vi "MatrixInit.vi"() -> ()   [LabVIEW 2026]
uses:
  <vilib>/MakerHub/LINX/Private/Type Defs/Peripherals/SPI/SPI Configuration.ctl
  <vilib>/MakerHub/LINX/Private/Type Defs/Peripherals/SPI/SPI Bit Order.ctl
  <vilib>/MakerHub/LINX/Private/Type Defs/Peripherals/SPI/SPI Mode.ctl
  <vilib>/MakerHub/LINX/Public/Peripherals/SPI/SPI Write Read N Frames.vi
  <vilib>/MakerHub/LINX/Private/Local IO/LinxSpiWriteRead.vi
  <vilib>/MakerHub/LINX/Public/Utilities/Check Channel.vi
  <vilib>/MakerHub/LINX/Private/Utilties/Generate Error.vi
  <vilib>/MakerHub/LINX/Public/Utilities/Open Serial.vi
  <vilib>/MakerHub/LINX/LMH-LINX.lvlib
  <vilib>/MakerHub/LINX/Private/Type Defs/Peripherals/SPI/SPI CS Logic Level.ctl
  <vilib>/MakerHub/LINX/Public/Peripherals/SPI/SPI CS Config.ctl
panel:
  in  "CS Configuration":T1
  out "Data":u8
  out "Address":u8
  out "Array 2":u8[](array[numeric])
  in  "Array":bool[][](array[boolean])
  in  "Stop Button":bool
  in  "SPI Configuration":T3={"Clock Frequency"=1000000, "Bit Order"=enum."LSb First", "SPI Mode"=enum."Mode 0"}
  in  "Serial Port":refnum<visa-resource-name>="N/A"
  # "Default 1000000 Hz"
  # "MAX7219 Matrix requires Most Significant Bit (MSb)!"
  # "Specify CS Pin on Arduino (10 in our setup)"
  # "MAX7219 requires Active Low Chip Select!"
  # "Just for debugging purposes!"
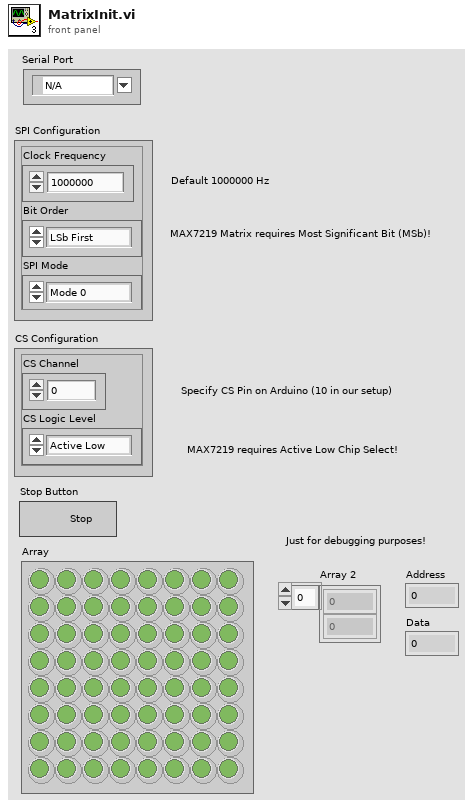
[diagram p1: front panel]
types:
  T1 = typedef "LMH-LINX.lvlib/SPI CS Config.ctl" = cluster{"CS Channel":u8, "CS Logic Level":T2}
  T2 = typedef "LMH-LINX.lvlib/SPI CS Logic Level.ctl" = enum8{"Active Low", "Active High"}
  T3 = typedef "LMH-LINX.lvlib/SPI Configuration.ctl" = cluster{"Clock Frequency":u32, "Bit Order":T4, "SPI Mode":T5}
  T4 = typedef "LMH-LINX.lvlib/SPI Bit Order.ctl" = enum8{"LSb First", "MSb First"}
  T5 = typedef "LMH-LINX.lvlib/SPI Mode.ctl" = enum8{"Mode 0", "Mode 1", "Mode 2", "Mode 3"}
  T6 = typedef "LMH-LINX.lvlib/LINX Ref.ctl" = cluster{"IO":T7, "Interface":T8, "LINX Device Config":T9}
  T7 = typedef "LMH-LINX.lvlib/Platform.ctl" = enum16{"Remote", "Local"}
  T8 = typedef "LMH-LINX.lvlib/Interface.ctl" = enum16{"Serial", "TCP"}
  T9 = typedef "LMH-LINX.lvlib/Device.lvlib/LINX Device Config.ctl" = cluster{"Interface":T8, "COM Port":refnum<visa-resource-name>, "TCP Configuration":T10, "Device Family":u8, "Device ID":u8, "Device Name":string, "TCP Ref":refnum<k5>, "Channels":T11}
  T10 = typedef "LMH-LINX.lvlib/Device.lvlib/TCP Config.ctl" = cluster{"IP Address":string, "Port":u16}
  T11 = typedef "LMH-LINX.lvlib/Channels.ctl" = cluster{"DI":u8[], "DO":u8[], "AI":u8[], "AO":u8[], "PWM":u8[], "QE":u8[], "UART":u8[], "I2C 2":u8[], "SPI":u8[], "CAN":u8[], "Servo":u8[], "AI Ref (V)":dbl, "AI Resolution (Bits)":u8, "AO Ref (V)":dbl, "AO Resolution (Bits)":u8}
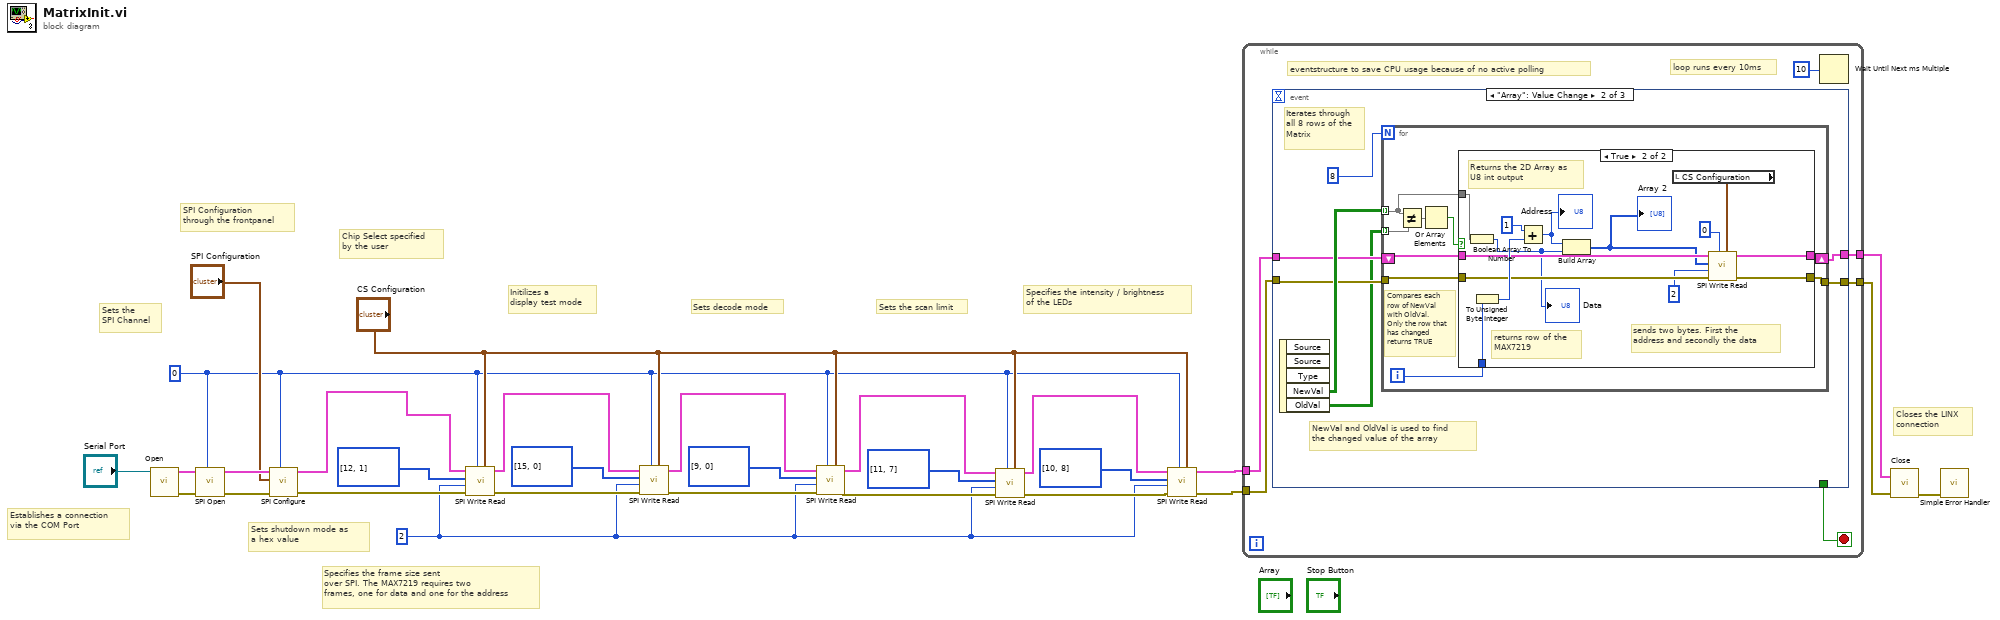
[diagram p0: block diagram]
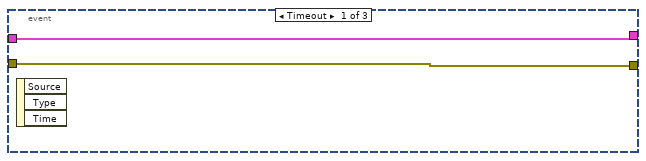
[diagram p2: hidden frame]
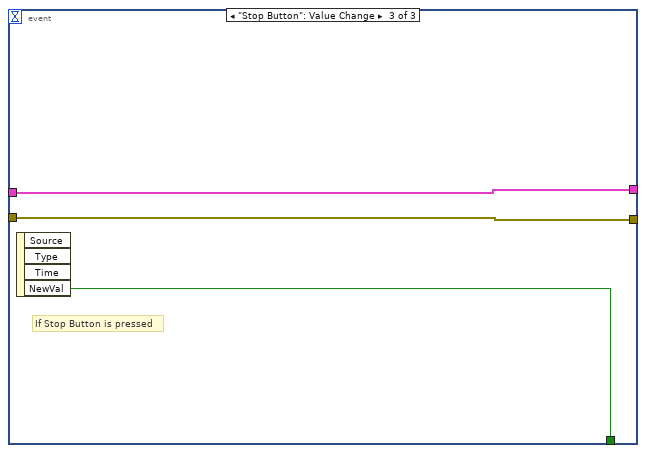
[diagram p4: hidden frame]
diagram:
  w2 = u8 2 ("SPI Frame Size")
  w1 = u8 0 ("SPI Channel (0)")
  # "Closes the LINX\nconnection"
  # "Specifies the intensity / brightness\nof the LEDs"
  # "Sets the scan limit"
  # "Sets decode mode"
  # "Initilizes a\ndisplay test mode"
  # "Sets shutdown mode as \na hex value"
  # "Specifies the frame size sent\nover SPI. The MAX7219 requires two\nframes, one for data and one for the address"
  # "Chip Select specified\nby the user"
  # "SPI Configuration\nthrough the frontpanel"
  # "Establishes a connection via the COM Port"
  # "Sets the\nSPI Channel"
  n1 = call-poly <vilib>:"Open.vi"("Serial Port"="Serial Port") -> ("Error Out"=w26:errorcluster, "LINX Resource"=w27:T6)  [unwired: 8 in, 1 out]
  n2 = call <vilib>:"SPI Open.vi"("SPI Channel (0)"=w1, "Error In"=w26, "LINX Resource"=w27) -> ("Error Out"=w24:errorcluster, "LINX Resource"=w25:T6)  [unwired: 7 in]
  n3 = call <vilib>:"SPI Configure.vi"("SPI Channel (0)"=w1, "Error In"=w24, "SPI Configuration"="SPI Configuration", "LINX Resource"=w25) -> ("Error Out"=w4:errorcluster, "LINX Resource"=w3:T6)  [unwired: 5 in, 1 out]
  n4 = call-poly <vilib>:"SPI Write Read.vi"("CS Configuration"="CS Configuration", "SPI Channel (0)"=w1, "Error In"=w4, "SPI Frame Size"=w2, "Data"=u8[] [12, 1], "LINX Resource"=w3) -> ("Error Out"=w15:errorcluster, "LINX Resource"=w14:T6)  [unwired: 2 in, 2 out]
  n5 = call-poly <vilib>:"SPI Write Read.vi"("CS Configuration"="CS Configuration", "SPI Channel (0)"=w1, "Error In"=w15, "SPI Frame Size"=w2, "Data"=u8[] [15, 0], "LINX Resource"=w14) -> ("Error Out"=w13:errorcluster, "LINX Resource"=w12:T6)  [unwired: 2 in, 2 out]
  n6 = call-poly <vilib>:"SPI Write Read.vi"("CS Configuration"="CS Configuration", "SPI Channel (0)"=w1, "Error In"=w13, "SPI Frame Size"=w2, "Data"=u8[] [9, 0], "LINX Resource"=w12) -> ("Error Out"=w10:errorcluster, "LINX Resource"=w11:T6)  [unwired: 2 in, 2 out]
  n7 = call-poly <vilib>:"SPI Write Read.vi"("CS Configuration"="CS Configuration", "SPI Channel (0)"=w1, "Error In"=w10, "SPI Frame Size"=w2, "Data"=u8[] [11, 7], "LINX Resource"=w11) -> ("Error Out"=w8:errorcluster, "LINX Resource"=w9:T6)  [unwired: 2 in, 2 out]
  n8 = call-poly <vilib>:"SPI Write Read.vi"("CS Configuration"="CS Configuration", "SPI Channel (0)"=w1, "Error In"=w8, "SPI Frame Size"=w2, "Data"=u8[] [10, 8], "LINX Resource"=w9) -> ("Error Out"=w6:errorcluster, "LINX Resource"=w5:T6)  [unwired: 2 in, 2 out]
  n9 = while {
    tunnel: w6 -> [w32]
    tunnel: w5 -> [w34]
    tunnel: [w33] -> w22
    tunnel: [w31] -> w21
    stop <- w30 stop-if-true
    # "loop runs every 10ms"
    # "eventstructure to save CPU usage because of no active polling"
    n10 = event shown="[1] \"Array\": Value Change" {
      selector: _ -> [_ _ _]
      dyn-events: _ -> [_ _ _]
      timeout: _ -> [_ _ _]
      tunnel: w34 -> [w37 w43 w72]
      tunnel: [w37 w42 w72] -> w33
      tunnel: w32 -> [w36 w41 w71]
      tunnel: [w36 w40 w71] -> w31
      tunnel: [_ _ w70] -> w30
      event Timeout {
        n11 = event-data() -> ()  [unwired: 1 in, 3 out]
      }
      event "Array": Value Change {
        # "Iterates through\nall 8 rows of the\nMatrix"
        # "NewVal and OldVal is used to find\nthe changed value of the array"
        n12 = event-data() -> ("NewVal"=w44:bool[][], "OldVal"=w38:bool[][])  [unwired: 1 in, 3 out]
        n13 = for {
          N: 8 -> [_]
          tunnel: w44 -> [w45] mode=indexing
          shift-right: [w50] -> w42
          shift-left: w43 -> [w52]
          tunnel: w41 -> [w51]
          tunnel: [w49] -> w40
          tunnel: w38 -> [w48] mode=indexing
          i -> [w53]
          # "Compares each row of NewVal with OldVal.\nOnly the row that has changed returns TRUE"
          n14 = Not Equal?(x=w45, y=w48) -> (x != y?=w47:bool[])
          n15 = Or Array Elements(Boolean array=w47) -> (logical OR=w46:bool)
          n16 = case shown="True" w46 {
            tunnel: w53 -> [_ w68]
            tunnel: w52 -> [w55 w64]
            tunnel: w51 -> [w54 w63]
            tunnel: [w55 w62] -> w50
            tunnel: [w54 w61] -> w49
            tunnel: w45 -> [_ w57]
            frame False {
            }
            frame True {
              # "returns row of the\nMAX7219"
              # "sends two bytes. First the\naddress and secondly the data"
              # "Returns the 2D Array as\nU8 int output"
              n17 = Boolean Array To Number(Boolean array=w57) -> (number=w58:u8)
              "Data" <- w58
              n18 = To Unsigned Byte Integer(number=w68) -> (unsigned 8bit integer=w67:u8)
              n19 = Add(x=u8 1 ("y"), y=w67) -> (x+y=w59:u8)
              "Address" <- w59
              n20 = Build Array(w59, w58) -> (w60:u8[])
              "Array 2" <- w60
              n21 = local read "CS Configuration"() -> (w65:T1)
              n22 = call-poly <vilib>:"SPI Write Read.vi"("CS Configuration"=w65, "SPI Channel (0)"=u8 0, "Error In"=w63, "SPI Frame Size"=u8 2, "Data"=w60, "LINX Resource"=w64) -> ("Error Out"=w61:errorcluster, "LINX Resource"=w62:T6)  [unwired: 2 in, 2 out]
            }
          }
        }
      }
      event "Stop Button": Value Change {
        # "If Stop Button is pressed"
        n23 = event-data() -> ("NewVal"=w70:bool)  [unwired: 1 in, 3 out]
      }
    }
    n24 = Wait Until Next ms Multiple(millisecond multiple=u32 10) -> ()  [unwired: 1 out]
  }
  n25 = call <vilib>:"Close.vi"("Error In"=w21, "LINX Resource"=w22) -> ("Error Out"=w28:errorcluster)  [unwired: 9 in]
  n26 = call <vilib>:"Simple Error Handler.vi"("error in (no error)"=w28) -> ()  [unwired: 4 in, 5 out]
